vi "Rabi-with-SPA.vi"() -> ()   [LabVIEW 2013]
uses:
  <vilib>/Analysis/NI_AALBase.lvlib
  <vilib>/Analysis/baseanly.llb/Mean (DBL).vi
panel:
  in  "GENERATOR":T1={"Gen Freq (Hz) "=3200000000.0, "Gen Power (dBm)"=10.0, "Generator Output"=FALSE, "address"="192.168.0.7"} {"Gen Power (dBm)" format="%#.3f"; "Gen Freq (Hz)" format="%^#.6e"}
  out "Expected time (h)":dbl
  in  "SPA":T2={"address"="192.168.0.6", "VBW (Hz)"=1000.0, "RBW (Hz)"=3000.0, "Span (Hz)"=20000000.0, "Points"=1001} {"Span (Hz)" format="%#.6p"; "RBW (Hz)" format="%#.6p"; "VBW (Hz)" format="%#.6p"}
  out "Time to wait (s)":dbl
  out "Measurment time (s)":dbl=0.493
  in  "Keysight":T3={"Keysight Connection"={"Type"=1, "VISA"="TCPIP0::192.168.0.8::inst0::INSTR", "GPIB"="10"}, "Frequency Parameters"={"Coupling"=TRUE, "Frequency 2 (MHz)"=2.0, "Frequency 1 (MHz)"=2.0, "WAVEFORM"=enum."PULSE"}, "Bucket pulse_width (ns)"=40.0, "Bucket pulse_delay (ns)"=65.0, "Start (ns)"=3.0, "End (ns)"=403.0, "Steps"=401} {"Frequency Parameters"."Frequency 1 (MHz)" min=0.0 max=14.5; "Frequency Parameters"."Frequency 2 (MHz)" min=0.0 max=14.5; "Keysight Connection"."Type" items=["VISA", "GPIB"]}
  out "Parameters":string
  out "Normalised":dbl[](graph)
  out "(Current)":i32=103
  in  "Averages":u32=1
  out "Total Background":dbl[][](graph)
  out "Total Signal":dbl[][](graph)
  out "(Current)":i32=103
  out "Background":dbl[](graph)
  out "Total Normalised Signal":dbl[][](graph)
  out "Signal":dbl[](graph)
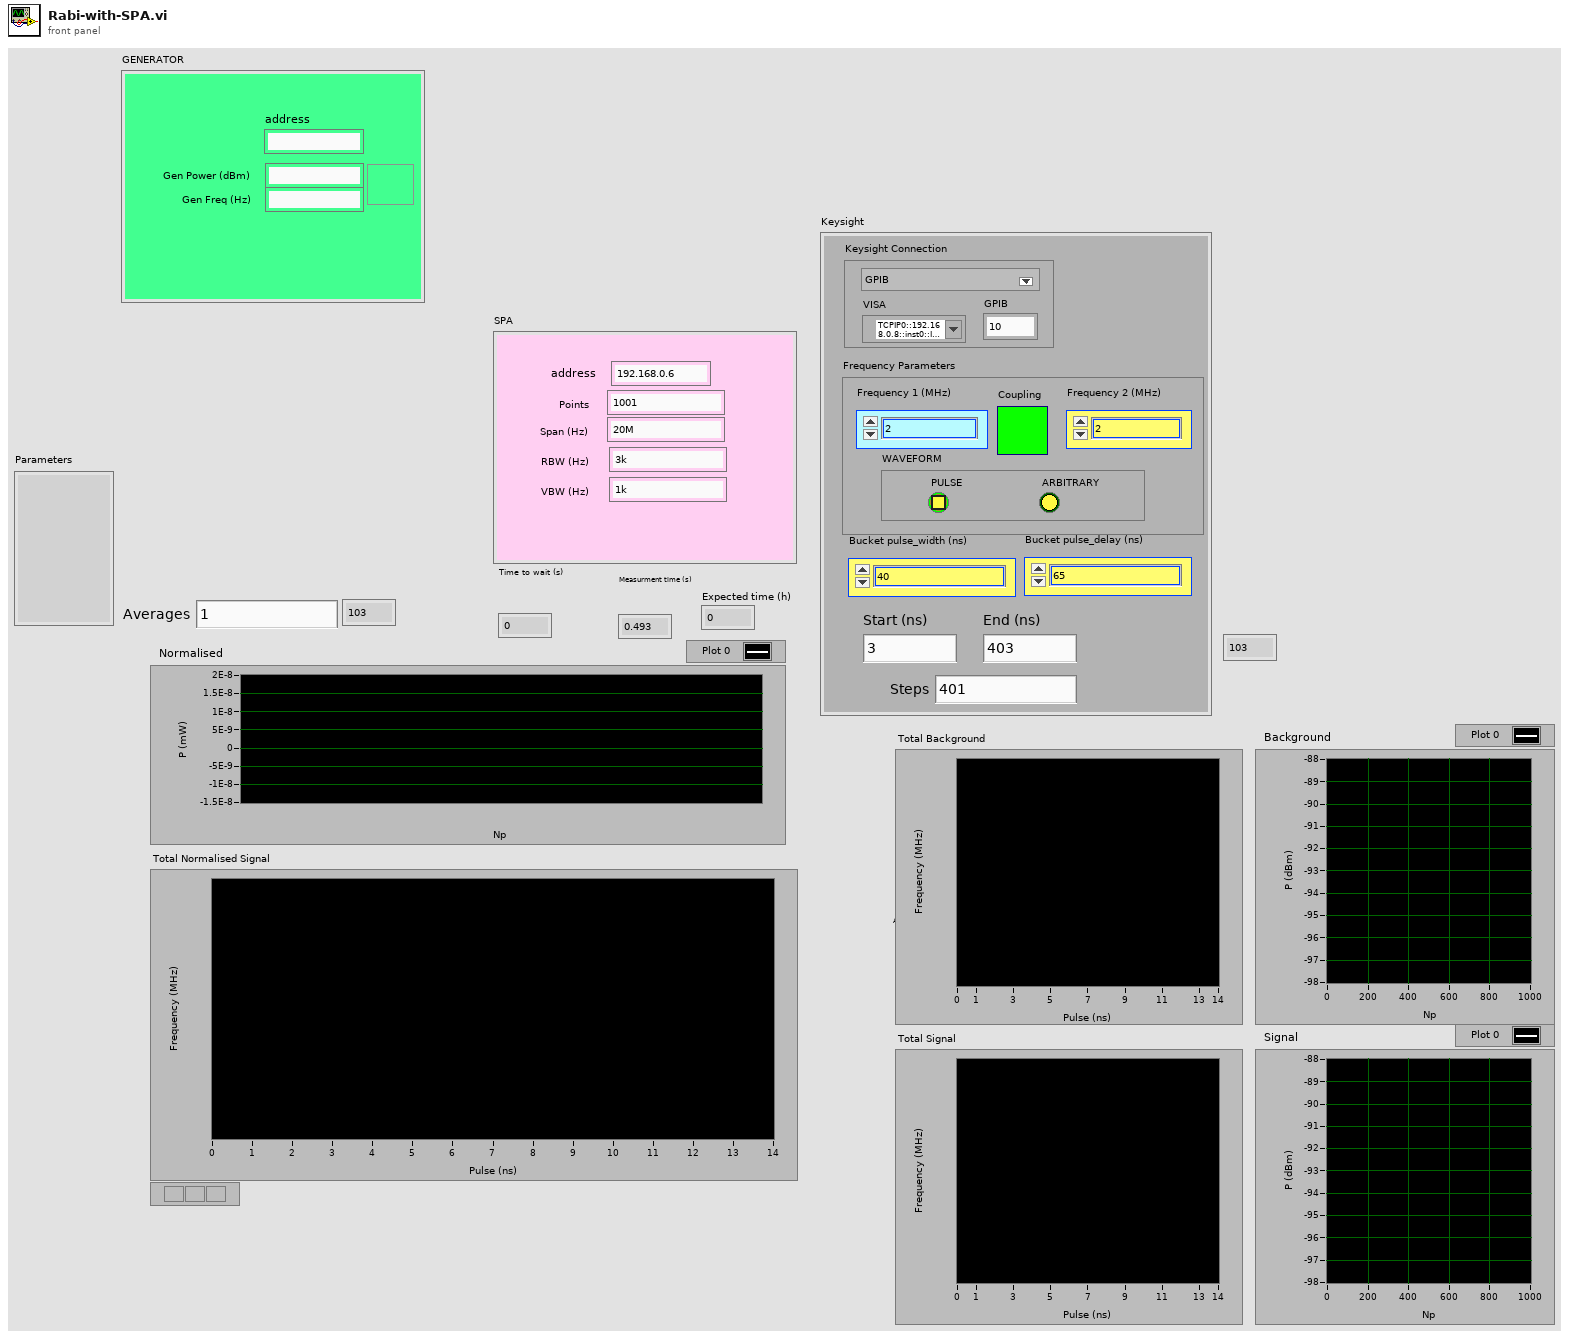
[diagram p1: front panel]
types:
  T1 = cluster{"Gen Freq (Hz) ":dbl, "Gen Power (dBm)":dbl, "Generator Output":bool, "address":string}
  T2 = cluster{"address":string, "VBW (Hz)":dbl, "RBW (Hz)":dbl, "Span (Hz)":dbl, "Points":i32}
  T3 = cluster{"Keysight Connection":cluster{"Type":u16, "VISA":refnum<visa-resource-name>, "GPIB":string}, "Frequency Parameters":cluster{"Coupling":bool, "Frequency 2 (MHz)":dbl, "Frequency 1 (MHz)":dbl, "WAVEFORM":enum32{"PULSE", "ARBITRARY"}}, "Bucket pulse_width (ns)":dbl, "Bucket pulse_delay (ns)":dbl, "Start (ns)":dbl, "End (ns)":dbl, "Steps":u32}
  T4 = cluster{"Ouput 1":bool, "Ouput 2":bool, "Ouput 1 Neg":bool, "Ouput 2 Neg":bool}
  T5 = cluster{"Type":u16, "VISA":refnum<visa-resource-name>, "GPIB":string}
  T6 = cluster{"Coupling":bool, "Frequency 2 (MHz)":dbl, "Frequency 1 (MHz)":dbl, "WAVEFORM":enum32{"PULSE", "ARBITRARY"}}
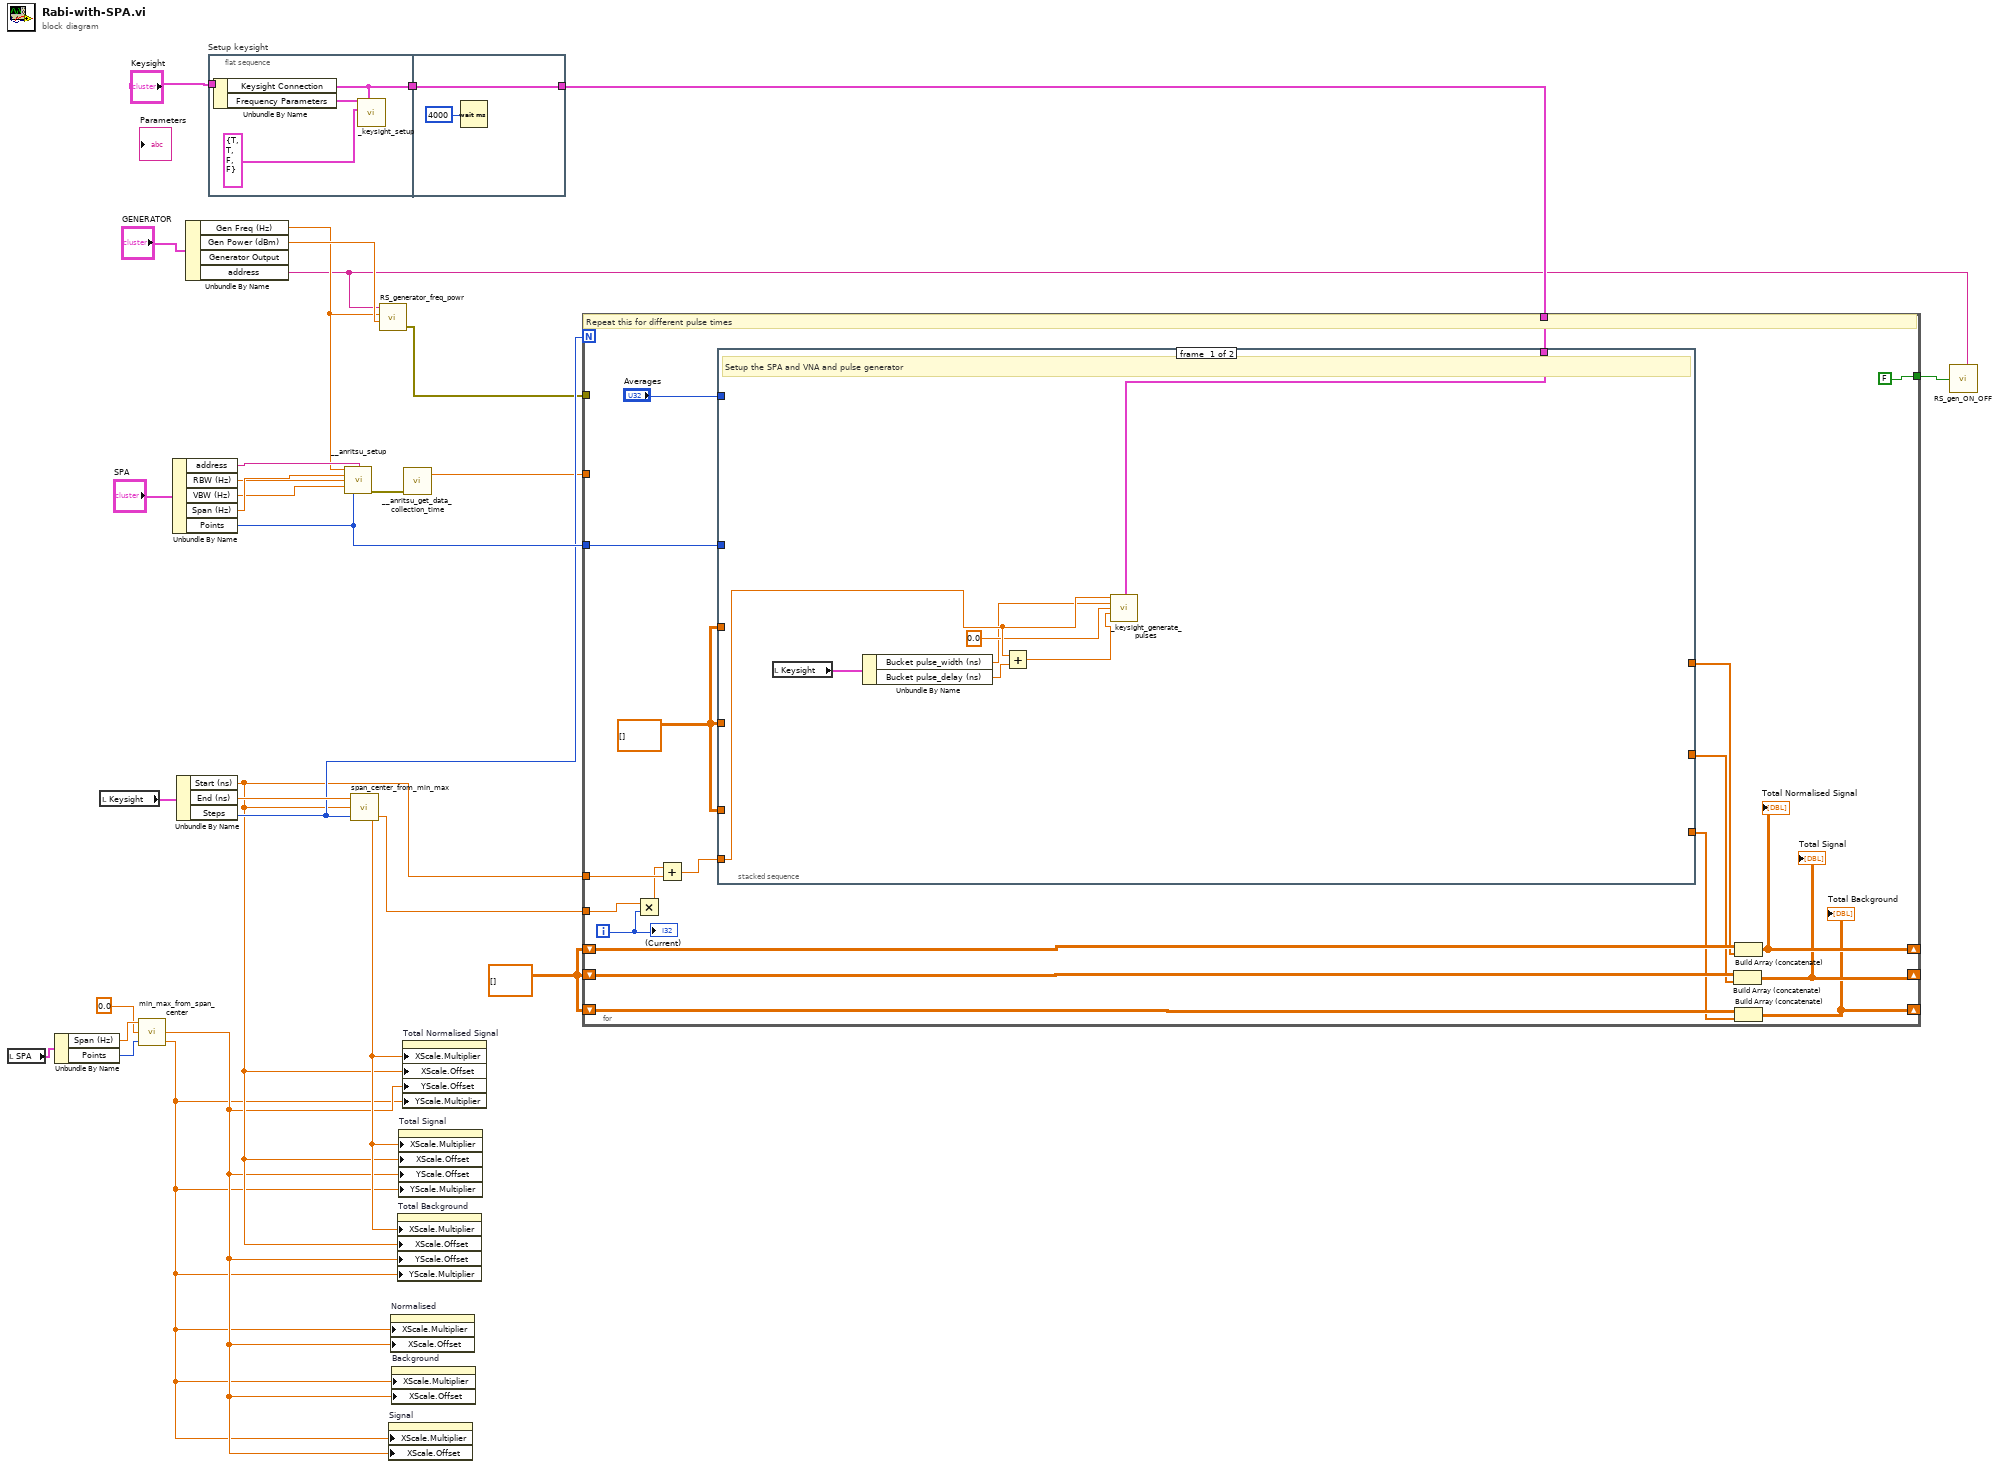
[diagram p0: block diagram]
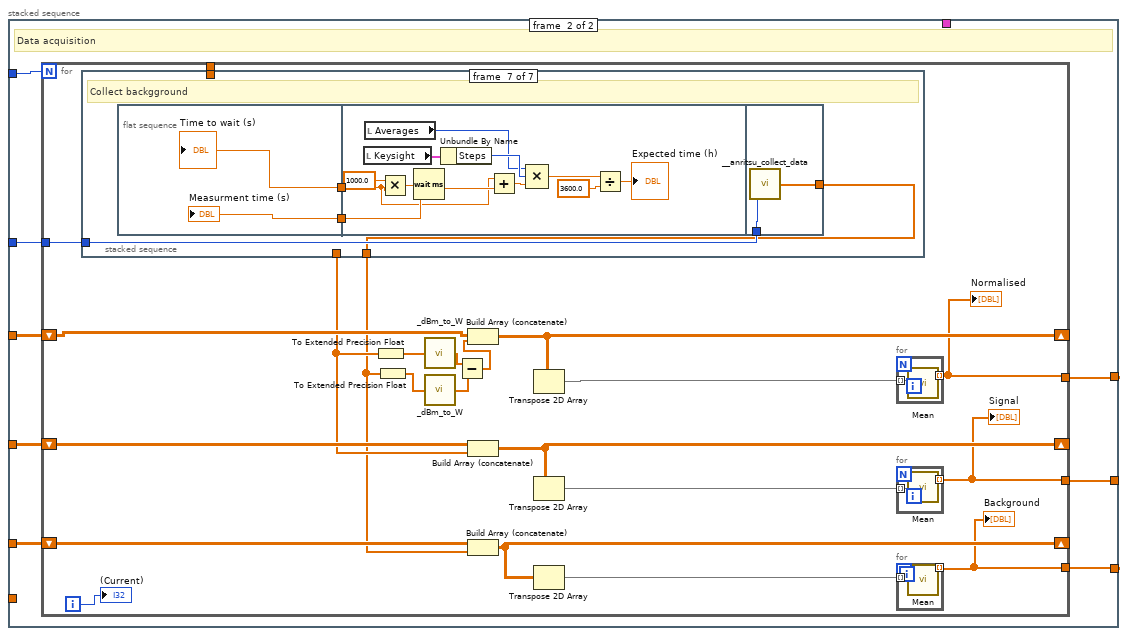
[diagram p2: hidden frame]
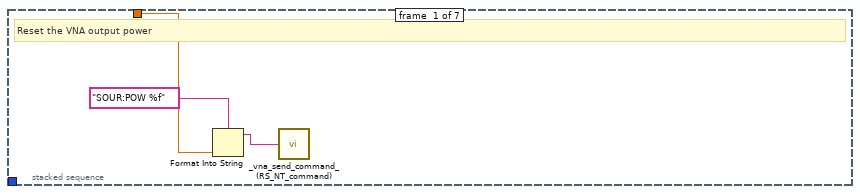
[diagram p3: hidden frame]
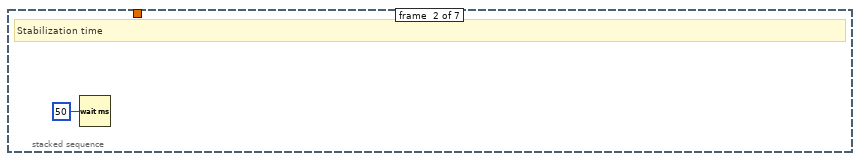
[diagram p4: hidden frame]
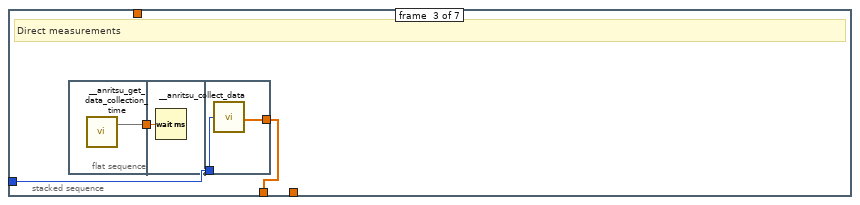
[diagram p5: hidden frame]
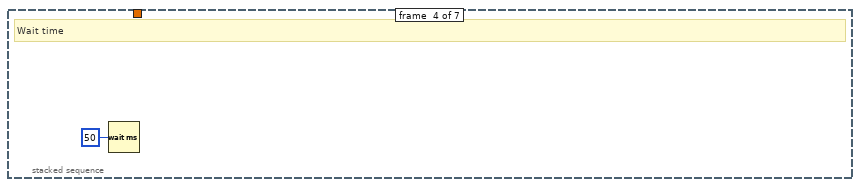
[diagram p6: hidden frame]
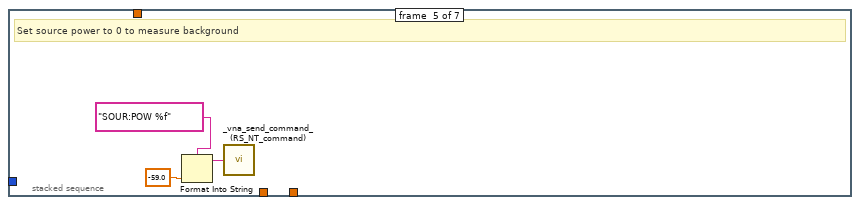
[diagram p7: hidden frame]
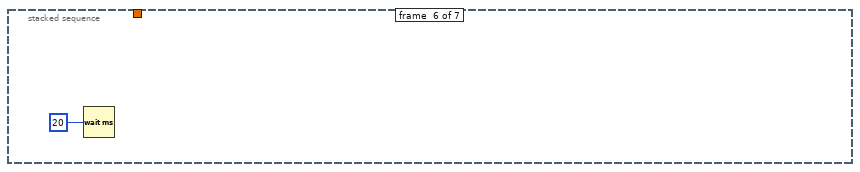
[diagram p8: hidden frame]
diagram:
  w29 = dbl[][] [] ("initialized array")
  n1 = local read "SPA"() -> (w16:T2)
  n2 = Unbundle By Name(w16) -> ("Span (Hz)"=w14:dbl, "Points"=w15:i32)
  n3 = local read "Keysight"() -> (w2:T3)
  n4 = call "min_max_from_span_center.vi"("No Points"=w15, "Mid Point"=0.0, "Span"=w14) -> ("Step"=w11:dbl, "Start"=w12:dbl)  [unwired: 1 out]
  n5 = Unbundle By Name("SPA") -> ("address"=w23:string, "RBW (Hz)"=w18:dbl, "VBW (Hz)"=w17:dbl, "Span (Hz)"=w21:dbl, "Points"=w22:i32)
  n6 = Unbundle By Name(w2) -> ("Start (ns)"=w19:dbl, "End (ns)"=w25:dbl, "Steps"=w20:u32)
  n7 = Unbundle By Name("GENERATOR") -> ("Gen Freq (Hz)"=w5:dbl, "Gen Power (dBm)"=w6:dbl, "address"=w4:string)  [unwired: 1 out]
  n8 = flat-sequence "Setup keysight" {
    tunnel: [w31] -> w26
    tunnel: "Keysight" -> [w32]
    tunnel: [w34] -> w27
    tunnel: w26 -> [w34]
    frame #0 {
      n9 = Unbundle By Name(w32) -> ("Keysight Connection"=w31:T5, "Frequency Parameters"=w30:T6)
      n10 = call "_keysight_setup.vi"("Frequency Parameters"=w30, "Outputs"=T4 {"Ouput 1"=TRUE, "Ouput 2"=TRUE, "Ouput 1 Neg"=FALSE, "Ouput 2 Neg"=FALSE}, "Keysight Connection"=w31) -> ()  [unwired: 3 in, 1 out]
    }
    frame #1 {
      n11 = Wait (ms)(milliseconds to wait=u32 4000) -> ()  [unwired: 1 out]
    }
  }
  n12 = call "__anritsu_setup.vi"("Center Freq (Hz)"=w5, "Points"=w22, "address"=w23, "Span (Hz)"=w21, "RBW (Hz)"=w18, "VBW (Hz)"=w17) -> ("error out"=w10:errorcluster)  [unwired: 8 in, 1 out]
  n13 = call "span_center_from_min_max.vi"("No Points"=w20, "Begin"=w19, "End"=w25) -> ("Step"=w28:dbl)  [unwired: 2 out]
  n14 = call "RS_generator_freq_powr.vi"("Power (dBm)"=w6, "Frequnecy (Hz)"=w5, "address"=w4) -> ("error out"=w3:errorcluster)  [unwired: 1 in, 2 out]
  n15 = property on="Signal" class="WFGraph (strict)"("XScale.Multiplier"=w11, "XScale.Offset"=w12) -> ()  [unwired: 2 in, 2 out]
  n16 = property on="Normalised" class="WFGraph (strict)"("XScale.Multiplier"=w11, "XScale.Offset"=w12) -> ()  [unwired: 2 in, 2 out]
  n17 = property on="Background" class="WFGraph (strict)"("XScale.Multiplier"=w11, "XScale.Offset"=w12) -> ()  [unwired: 2 in, 2 out]
  n18 = property on="Total Background" class="IntGraph (strict)"("XScale.Multiplier"=w28, "XScale.Offset"=w19, "YScale.Offset"=w12, "YScale.Multiplier"=w11) -> ()  [unwired: 2 in, 2 out]
  n19 = property on="Total Signal" class="IntGraph (strict)"("XScale.Multiplier"=w28, "XScale.Offset"=w19, "YScale.Offset"=w12, "YScale.Multiplier"=w11) -> ()  [unwired: 2 in, 2 out]
  n20 = property on="Total Normalised Signal" class="IntGraph (strict)"("XScale.Multiplier"=w28, "XScale.Offset"=w19, "YScale.Offset"=w12, "YScale.Multiplier"=w11) -> ()  [unwired: 2 in, 2 out]
  n21 = call "__anritsu_get_data_collection_time.vi"("error in"=w10) -> ("Measurment time (s)"=w9:dbl)  [unwired: 1 in, 1 out]
  n22 = for {
    N: w20 -> [_]
    shift-right: [w51] -> _
    shift-left: w29 -> [w53]
    tunnel: w28 -> [w40]
    tunnel: w19 -> [w42]
    shift-right: [w46] -> _
    shift-left: w29 -> [w50]
    shift-right: [w45] -> _
    shift-left: w29 -> [w49]
    tunnel: w22 -> [w38]
    tunnel: w27 -> [w37]
    tunnel: w9 -> [_]
    tunnel: [FALSE ("Generator Output")] -> w7
    tunnel: w3 -> [_]
    i -> [w41]
    w44 = dbl[][] [] ("initialized array")
    # "Repeat this for different pulse times"
    n23 = Multiply(x=w40, y=w41) -> (x*y=w39:dbl)
    n24 = Add(x=w39, y=w42) -> (x+y=w43:dbl)
    n25 = stacked-sequence {
      tunnel: "Averages" -> [_ w70]
      tunnel: [_ w69] -> w52
      tunnel: [_ w68] -> w48
      tunnel: [_ w67] -> w47
      tunnel: w44 -> [_ w66]
      tunnel: w44 -> [_ w65]
      tunnel: w44 -> [_ w64]
      tunnel: w43 -> [w61 _]
      tunnel: w38 -> [_ w63]
      tunnel: w37 -> [w60 _]
      frame #0 {
        # "Setup the SPA and VNA and pulse generator"
        n26 = local read "Keysight"() -> (w57:T3)
        n27 = Unbundle By Name(w57) -> ("Bucket pulse_width (ns)"=w55:dbl, "Bucket pulse_delay (ns)"=w56:dbl)
        n28 = Add(x=w61, y=w56) -> (x+y=w58:dbl)
        n29 = call "_keysight_generate_pulses.vi"("Ch1 pulse_width (ns)"=w61, "Connection"=w60, "Ch2 pulse_width (ns)"=w55, "Ch1 pulse_delay (ns)"=0.0 ("Ch2 pulse_delay (ns)"), "Ch2 pulse_delay (ns)"=w58) -> ()  [unwired: 9 in, 2 out]
      }
      frame #1 {
        # "Data acquisition"
        n30 = for {
          N: w70 -> [_]
          shift-right: [w80] -> _
          shift-left: w66 -> [w92]
          tunnel: [w78] -> w69
          shift-right: [w85] -> _
          shift-left: w65 -> [w89]
          shift-right: [w84] -> _
          shift-left: w64 -> [w88]
          tunnel: [w77] -> w68
          tunnel: [w76] -> w67
          tunnel: w63 -> [w83]
          tunnel: [w79] -> w62
          i -> [w90]
          n31 = stacked-sequence {
            tunnel: [_ _ w103 _ _ _ _] -> w82
            tunnel: [_ _ _ _ _ _ w116] -> w81
            tunnel: w83 -> [_ _ w105 _ _ _ w118]
            tunnel: w79 -> [w99 _ _ _ _ _ _]
            frame #0 {
              # "Reset the VNA output power"
              n32 = Format Into String(format string="SOUR:POW %f" ("Comand"), w99) -> (resulting string=w100:string)  [unwired: 2 in, 1 out]
              n33 = call "_vna_send_command_(RS_NT_command).vi"("Comand"=w100) -> ()  [unwired: 4 in, 1 out]
            }
            frame #1 {
              # "Stabilization time"
              n34 = Wait (ms)(milliseconds to wait=u32 50) -> ()  [unwired: 1 out]
            }
            frame #2 {
              # "Direct measurements"
              n35 = flat-sequence {
                tunnel: [w106] -> w104
                tunnel: w104 -> [w107]
                tunnel: [w109] -> w103
                tunnel: w105 -> [w108]
                frame #0 {
                  n36 = call "__anritsu_get_data_collection_time.vi"() -> (1:w106)  [unwired: 1 out]
                }
                frame #1 {
                  n37 = Wait (ms)(milliseconds to wait=w107) -> ()  [unwired: 1 out]
                }
                frame #2 {
                  n38 = call "__anritsu_collect_data.vi"("Points to read"=w108) -> ("Data out"=w109:dbl[])
                }
              }
            }
            frame #3 {
              # "Wait time"
              n39 = Wait (ms)(milliseconds to wait=u32 50) -> ()  [unwired: 1 out]
            }
            frame #4 {
              # "Set source power to 0 to measure background"
              n40 = Format Into String(format string="SOUR:POW %f" ("Comand"), -59.0 ("input 2")) -> (resulting string=w112:string)  [unwired: 2 in, 1 out]
              n41 = call "_vna_send_command_(RS_NT_command).vi"("Comand"=w112) -> ()  [unwired: 4 in, 1 out]
            }
            frame #5 {
              n42 = Wait (ms)(milliseconds to wait=u32 20) -> ()  [unwired: 1 out]
            }
            frame #6 {
              # "Collect backgground"
              n43 = flat-sequence {
                tunnel: [w120] -> w117
                tunnel: ["Measurment time (s)"] -> w115
                tunnel: w117 -> [w123]
                tunnel: w115 -> [w130]
                tunnel: w118 -> [w133]
                tunnel: [w132] -> w116
                frame #0 {
                  "Time to wait (s)" <- w120
                }
                frame #1 {
                  n44 = local read "Keysight"() -> (w131:T3)
                  n45 = local read "Averages"() -> (w128:u32)
                  n46 = Multiply(x=1000.0, y=w123) -> (x*y=w121:dbl)
                  n47 = Wait (ms)(milliseconds to wait=w121) -> ()  [unwired: 1 out]
                  n48 = Unbundle By Name(w131) -> ("Steps"=w129:u32)
                  n49 = Add(x=w123, y=w130) -> (x+y=w127:dbl)
                  n50 = Compound Arithmetic op=MULTIPLY(w128, w129, w127) -> (w126:dbl)
                  n51 = Divide(x=w126, y=3600.0) -> (x/y=→"Expected time (h)":dbl)
                }
                frame #2 {
                  n52 = call "__anritsu_collect_data.vi"("Points to read"=w133) -> ("Data out"=w132:dbl[])
                }
              }
            }
          }
          n53 = To Extended Precision Float(1:w82) -> (0:w75:ext[])
          n54 = To Extended Precision Float(1:w81) -> (0:w74:ext[])
          n55 = call "_dBm_to_W.vi"("Power dBm"=w75) -> ("Power W"=w73:dbl[])
          n56 = call "_dBm_to_W.vi"("Power dBm"=w74) -> ("Power W"=w72:dbl[])
          n57 = Subtract(x=w73, y=w72) -> (x-y=w71:dbl[])
          n58 = Build Array (concatenate)(w92, w71) -> (w80:dbl[][])
          n59 = Build Array (concatenate)(w89, w82) -> (w85:dbl[][])
          n60 = Build Array (concatenate)(w88, w81) -> (w84:dbl[][])
          n61 = Transpose 2D Array(2D array=w80) -> (transposed array=w91:dbl[][])
          n62 = Transpose 2D Array(2D array=w85) -> (transposed array=w87:dbl[][])
          n63 = Transpose 2D Array(2D array=w84) -> (transposed array=w86:dbl[][])
          n64 = for {
            tunnel: w91 -> [w98] mode=indexing
            tunnel: [w97] -> w78 mode=indexing
            n65 = call-poly <vilib>:"Mean.vi"("X"=w98) -> ("mean"=w97:dbl)  [unwired: 1 out]
          }
          "Normalised" <- w78
          n66 = for {
            tunnel: w87 -> [w96] mode=indexing
            tunnel: [w95] -> w77 mode=indexing
            n67 = call-poly <vilib>:"Mean.vi"("X"=w96) -> ("mean"=w95:dbl)  [unwired: 1 out]
          }
          "Signal" <- w77
          n68 = for {
            tunnel: w86 -> [w94] mode=indexing
            tunnel: [w93] -> w76 mode=indexing
            n69 = call-poly <vilib>:"Mean.vi"("X"=w94) -> ("mean"=w93:dbl)  [unwired: 1 out]
          }
          "Background" <- w76
          "(Current)" <- w90
        }
      }
    }
    n70 = Build Array (concatenate)(w50, w48) -> (w46:dbl[][])
    "Total Signal" <- w46
    n71 = Build Array (concatenate)(w53, w52) -> (w51:dbl[][])
    "Total Normalised Signal" <- w51
    n72 = Build Array (concatenate)(w49, w47) -> (w45:dbl[][])
    "Total Background" <- w45
    "(Current)" <- w41
  }
  n73 = call "RS_gen_ON_OFF.vi"("Generator Output"=w7, "address"=w4) -> ()  [unwired: 3 in, 1 out]
